vi "display.vi"(11 "Array":T1(array[cluster])) -> ()   [LabVIEW 2014]
panel:
  in  "go to NO.":i32
  out "elecFee":dbl[][](graph)
  out "Total Number of Options":i32 caption="size(s)"
  in  "panel":T2
  out "LEDs elecFee (NTD/day)":dbl
  out "ACs elecFee (NTD/day)":dbl
  out "Total elecFee (NTD/day)":dbl
  out "Group 1":bool[](array[boolean])
  out "Group 2":bool[](array[boolean])
  out "Group 3":bool[](array[boolean])
  out "NO.":i32
  # "Lightening Arrange"
  # "2~3"
  # "0~1"
  # "1~2"
  # "3~4"
  # "4~5"
  # "5~6"
  # "6~7"
  # "7~8"
  # "8~9"
  # "9~10"
  # "10~11"
  # "11~12"
  # "12~13"
  # "13~14"
  # "14~15"
  # "15~16"
  # "16~17"
  # "17~18"
  # "18~19"
  # "19~20"
  # "21~21"
  # "21~22"
  # "22~23"
  # "23~24"
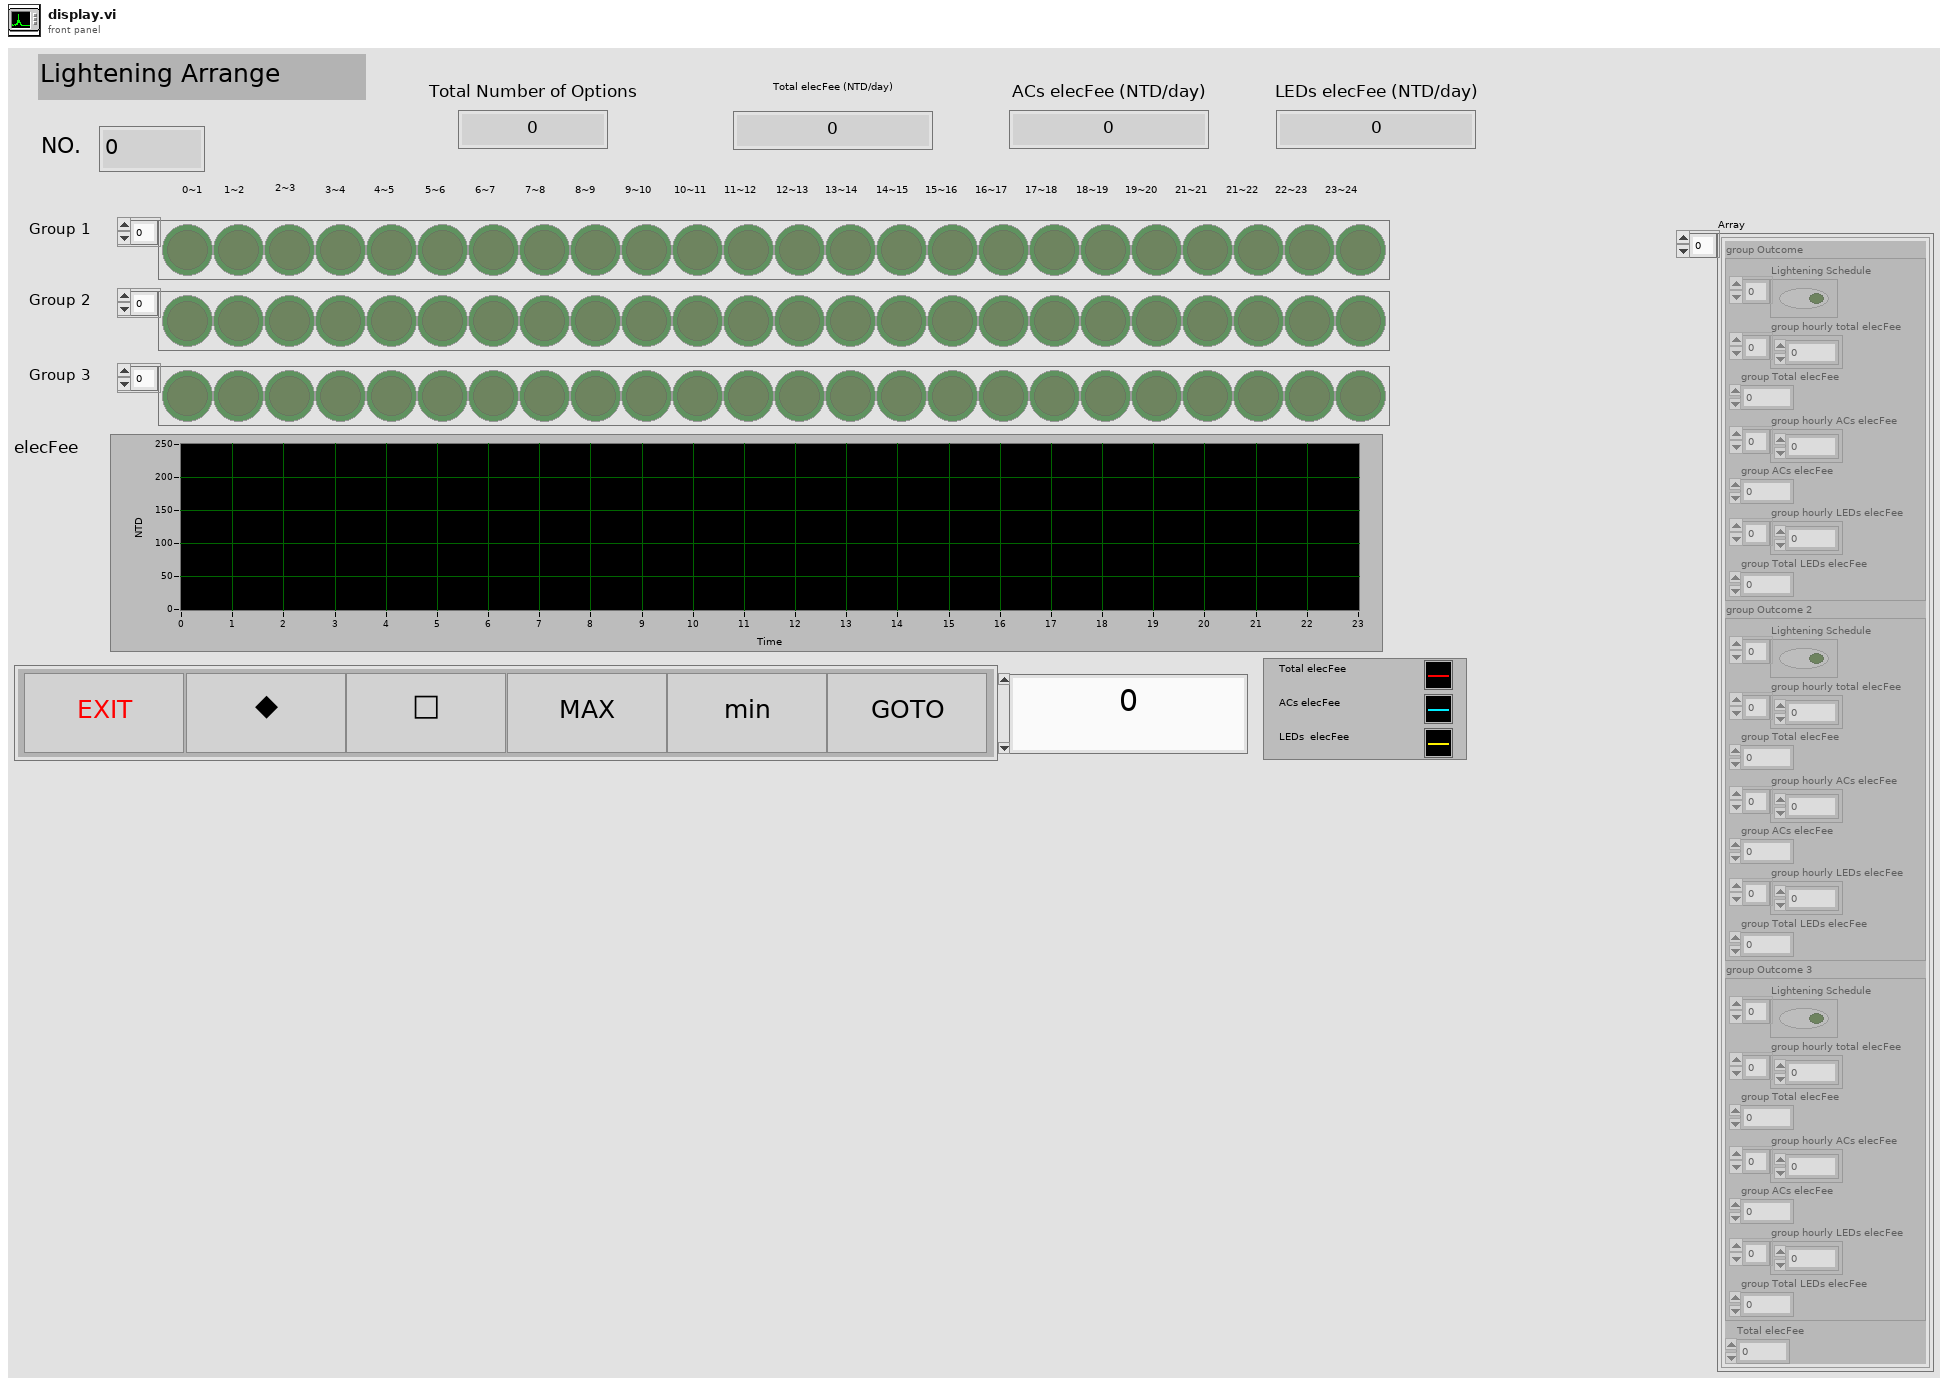
[diagram p1: front panel]
types:
  T1 = cluster{"group Outcome":cluster{"Lightening Schedule":bool[], "group hourly total elecFee":dbl[], "group Total elecFee":dbl, "group hourly ACs elecFee":dbl[], "group ACs elecFee":dbl, "group hourly LEDs elecFee":dbl[], "group Total LEDs elecFee":dbl}, "group Outcome 2":cluster{"Lightening Schedule":bool[], "group hourly total elecFee":dbl[], "group Total elecFee":dbl, "group hourly ACs elecFee":dbl[], "group ACs elecFee":dbl, "group hourly LEDs elecFee":dbl[], "group Total LEDs elecFee":dbl}, "group Outcome 3":cluster{"Lightening Schedule":bool[], "group hourly total elecFee":dbl[], "group Total elecFee":dbl, "group hourly ACs elecFee":dbl[], "group ACs elecFee":dbl, "group hourly LEDs elecFee":dbl[], "group Total LEDs elecFee":dbl}, "Total elecFee":dbl}[]
  T2 = cluster{"◆":bool, "□":bool, "MAX":bool, "min":bool, "EXIT":bool, "min 2":bool}
  T3 = cluster{"group Outcome":cluster{"Lightening Schedule":bool[], "group hourly total elecFee":dbl[], "group Total elecFee":dbl, "group hourly ACs elecFee":dbl[], "group ACs elecFee":dbl, "group hourly LEDs elecFee":dbl[], "group Total LEDs elecFee":dbl}, "group Outcome 2":cluster{"Lightening Schedule":bool[], "group hourly total elecFee":dbl[], "group Total elecFee":dbl, "group hourly ACs elecFee":dbl[], "group ACs elecFee":dbl, "group hourly LEDs elecFee":dbl[], "group Total LEDs elecFee":dbl}, "group Outcome 3":cluster{"Lightening Schedule":bool[], "group hourly total elecFee":dbl[], "group Total elecFee":dbl, "group hourly ACs elecFee":dbl[], "group ACs elecFee":dbl, "group hourly LEDs elecFee":dbl[], "group Total LEDs elecFee":dbl}, "Total elecFee":dbl}
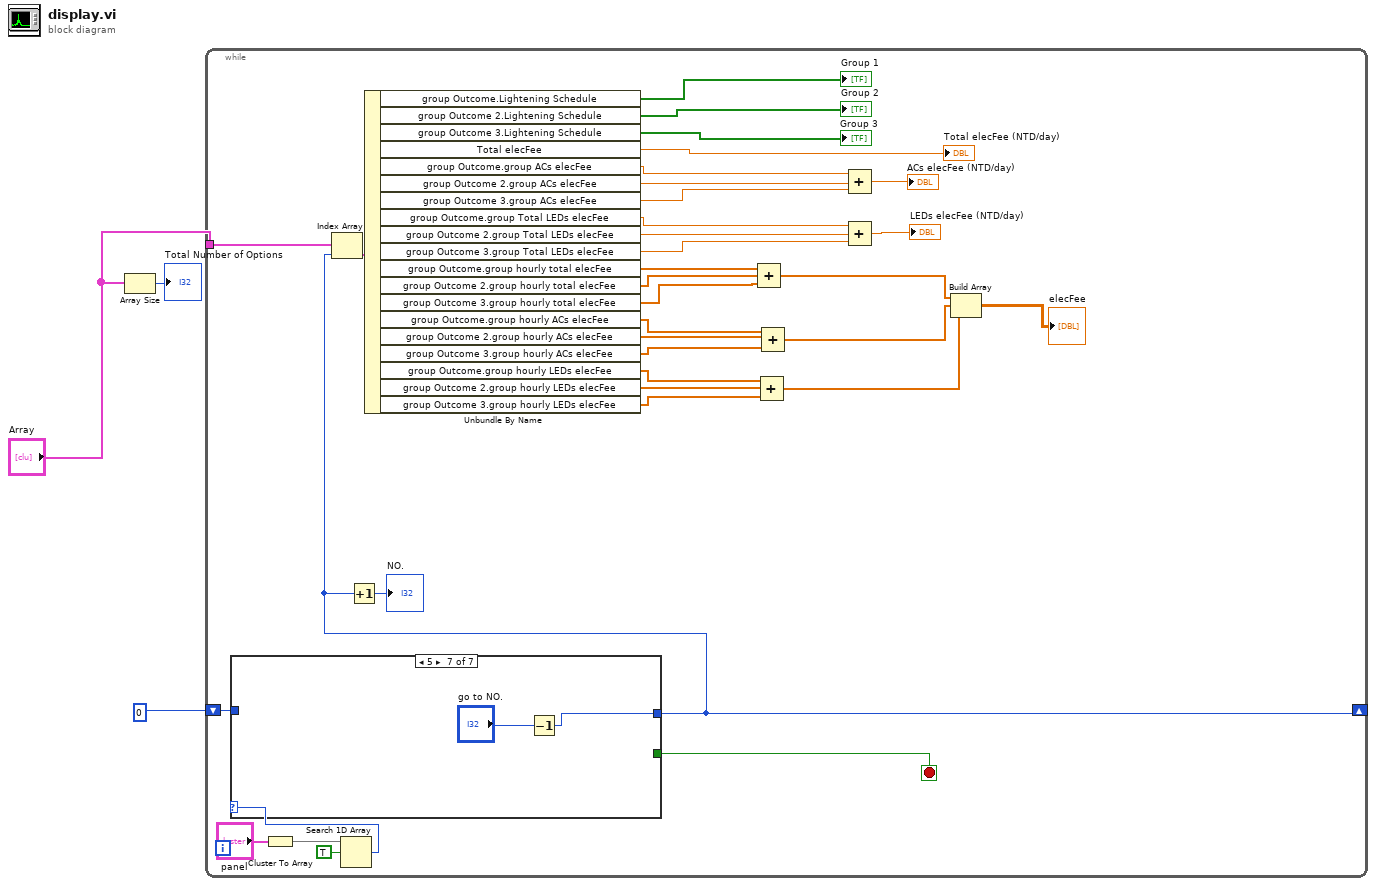
[diagram p0: block diagram]
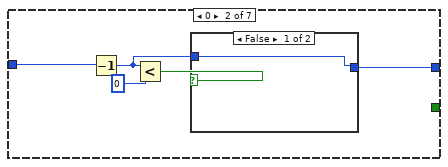
[diagram p3: hidden frame]
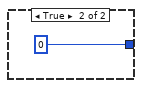
[diagram p4: hidden frame]
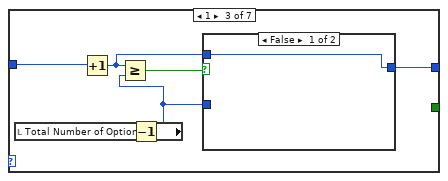
[diagram p5: hidden frame]
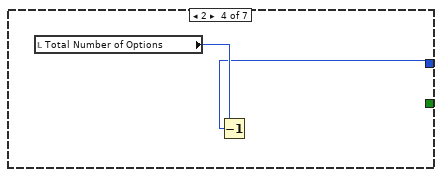
[diagram p7: hidden frame]
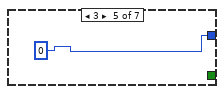
[diagram p8: hidden frame]
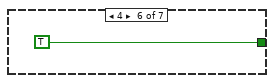
[diagram p9: hidden frame]
diagram:
  n1 = Array Size(array="Array") -> (size(s)=→"Total Number of Options":i32)
  n2 = while {
    tunnel: "Array" -> [w38]
    shift-right: [w4] -> _
    shift-left: 0 -> [w33]
    stop <- w19 stop-if-true
    n3 = Cluster To Array(cluster="panel") -> (array=w36:bool[])
    n4 = Search 1D Array(1D array=w36, element=TRUE) -> (index of element=w34:i32)  [unwired: 1 in]
    n5 = case shown="5" w34 {
      tunnel: w33 -> [w39 w44 w52 _ _ _ _]
      tunnel: [w39 w41 w48 w55 0 _ w60] -> w4
      tunnel: [_ _ _ _ _ TRUE _] -> w19
      frame -1, Default {
      }
      frame 0 {
        n6 = Decrement(x=w44) -> (x-1=w40:i32)
        n7 = Less?(x=w40, y=0) -> (x < y?=w42:bool)
        n8 = case shown="False" w42 {
          tunnel: [w45 0 ("y")] -> w41
          tunnel: w40 -> [w45 _]
          frame False {
          }
          frame True {
          }
        }
      }
      frame 1 {
        n9 = local read "Total Number of Options"() -> (w51:i32)
        n10 = Increment(x=w52) -> (x+1=w47:i32)
        n11 = Decrement(x=w51) -> (x-1=w49:i32)
        n12 = Greater Or Equal?(x=w47, y=w49) -> (x >= y?=w50:bool)
        n13 = case shown="False" w50 {
          tunnel: w49 -> [_ w54]
          tunnel: [w53 w54] -> w48
          tunnel: w47 -> [w53 _]
          frame False {
          }
          frame True {
          }
        }
      }
      frame 2 {
        n14 = local read "Total Number of Options"() -> (w56:i32)
        n15 = Decrement(x=w56) -> (x-1=w55:i32)
      }
      frame 3 {
      }
      frame 4 {
      }
      frame 5 {
        n16 = Decrement(x="go to NO.") -> (x-1=w60:i32)
      }
    }
    n17 = Index Array(array=w38, index=w4) -> (element=w32:T3)
    n18 = Increment(x=w4) -> (x+1=→"NO.":i32)
    n19 = Unbundle By Name(w32) -> ("group Outcome.Lightening Schedule"=→"Group 1":bool[], "group Outcome 2.Lightening Schedule"=→"Group 2":bool[], "group Outcome 3.Lightening Schedule"=→"Group 3":bool[], "Total elecFee"=→"Total elecFee (NTD/day)":dbl, "group Outcome.group ACs elecFee"=w31:dbl, "group Outcome 2.group ACs elecFee"=w30:dbl, "group Outcome 3.group ACs elecFee"=w29:dbl, "group Outcome.group Total LEDs elecFee"=w28:dbl, "group Outcome 2.group Total LEDs elecFee"=w27:dbl, "group Outcome 3.group Total LEDs elecFee"=w26:dbl, "group Outcome.group hourly total elecFee"=w18:dbl[], "group Outcome 2.group hourly total elecFee"=w17:dbl[], "group Outcome 3.group hourly total elecFee"=w16:dbl[], "group Outcome.group hourly ACs elecFee"=w15:dbl[], "group Outcome 2.group hourly ACs elecFee"=w14:dbl[], "group Outcome 3.group hourly ACs elecFee"=w13:dbl[], "group Outcome.group hourly LEDs elecFee"=w12:dbl[], "group Outcome 2.group hourly LEDs elecFee"=w11:dbl[], "group Outcome 3.group hourly LEDs elecFee"=w10:dbl[])
    n20 = Compound Arithmetic op=ADD(w18, w17, w16) -> (w9:dbl[])
    n21 = Compound Arithmetic op=ADD(w12, w11, w10) -> (w6:dbl[])
    n22 = Compound Arithmetic op=ADD(w15, w14, w13) -> (w7:dbl[])
    n23 = Compound Arithmetic op=ADD(w31, w30, w29) -> (→"ACs elecFee (NTD/day)":dbl)
    n24 = Compound Arithmetic op=ADD(w28, w27, w26) -> (→"LEDs elecFee (NTD/day)":dbl)
    n25 = Build Array(w9, w7, w6) -> (→"elecFee":dbl[][])
  }
